vi "SCMP - Set Exp and Check FPS.vi"(6 "Andor":T1={"Handle"=0, "Pixel Encoding"="", "AOI Width"=0, "AOI Height"=0, "AOI Stride"=0, "Row Readout Time"=0.0, "Frame Readout Time"=0.0, "Interframe Time"=0.0, "Semaphore"=refnum, "SerialNumber"="", "Camera Model"="", "Controller ID"="", "Firmware Version"="", "Shutter"="Global", "BDiv"=1, "Time at Synch"=timestamp(3029526000.379448 s since 1904-01-01), "Idx"=0, "PreAmp"="", "Binning"=enum."1x1", "PixelReadoutRate"="", "Exposure (s)"=0.05, "Image Bytes"=0, "Image Pixels"=0, "SpuriousNoiseFilter"=FALSE, "Overlap"=FALSE, "CycleMode"=""} {"Exposure (s)" format="%^.3g"; "Time at Synch" format="%<%H:%M:%S>T"; "Interframe Time" format="%#_3g"; "Frame Readout Time" format="%_3g"; "Row Readout Time" format="%_3g"}, 7 "Set Exp or Check Fps (Set Exp)":enum16{"Set Exp", "Check FPS"}(ring), 8 "error in (no error)":errorcluster, 11 "Exposure [s]":dbl) -> (0 "error out":errorcluster, 3 "FPS":dbl=1.0)   [LabVIEW 2014]
doc: "Use this template to build a VI to use as a subVI."
uses:
  Camera/Andor Neo Info.ctl
  Controls/beaning.ctl
panel:
  out "FPS out":dbl=25.0 format="%.2f"
  out "Is Camera Exposure Acceptable":bool
  out "Maximum Exposure [ms]":dbl
  in  "FPS in":dbl=25.0 format="%0.2p"
  # "disabled"
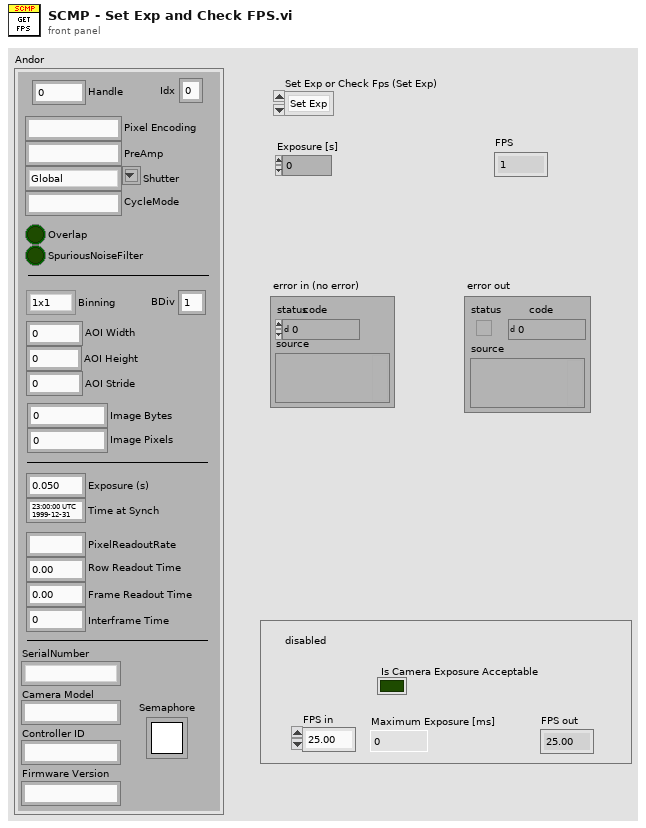
[diagram p1: front panel]
types:
  T1 = typedef "Andor Neo Info.ctl" = cluster{"Handle":i32, "Pixel Encoding":string, "AOI Width":i32, "AOI Height":i32, "AOI Stride":i32, "Row Readout Time":dbl, "Frame Readout Time":dbl, "Interframe Time":dbl, "Semaphore":T2, "SerialNumber":string, "Camera Model":string, "Controller ID":string, "Firmware Version":string, "Shutter":string, "BDiv":u8, "Time at Synch":timestamp, "Idx":i32, "PreAmp":string, "Binning":T3, "PixelReadoutRate":string, "Exposure (s)":dbl, "Image Bytes":i64, "Image Pixels":i64, "SpuriousNoiseFilter":bool, "Overlap":bool, "CycleMode":string}
  T2 = typedef "Semaphore RefNum" = refnum<k1>
  T3 = typedef "beaning.ctl" = enum16{"1x1", "2x2", "3x3", "4x4", "8x8"}
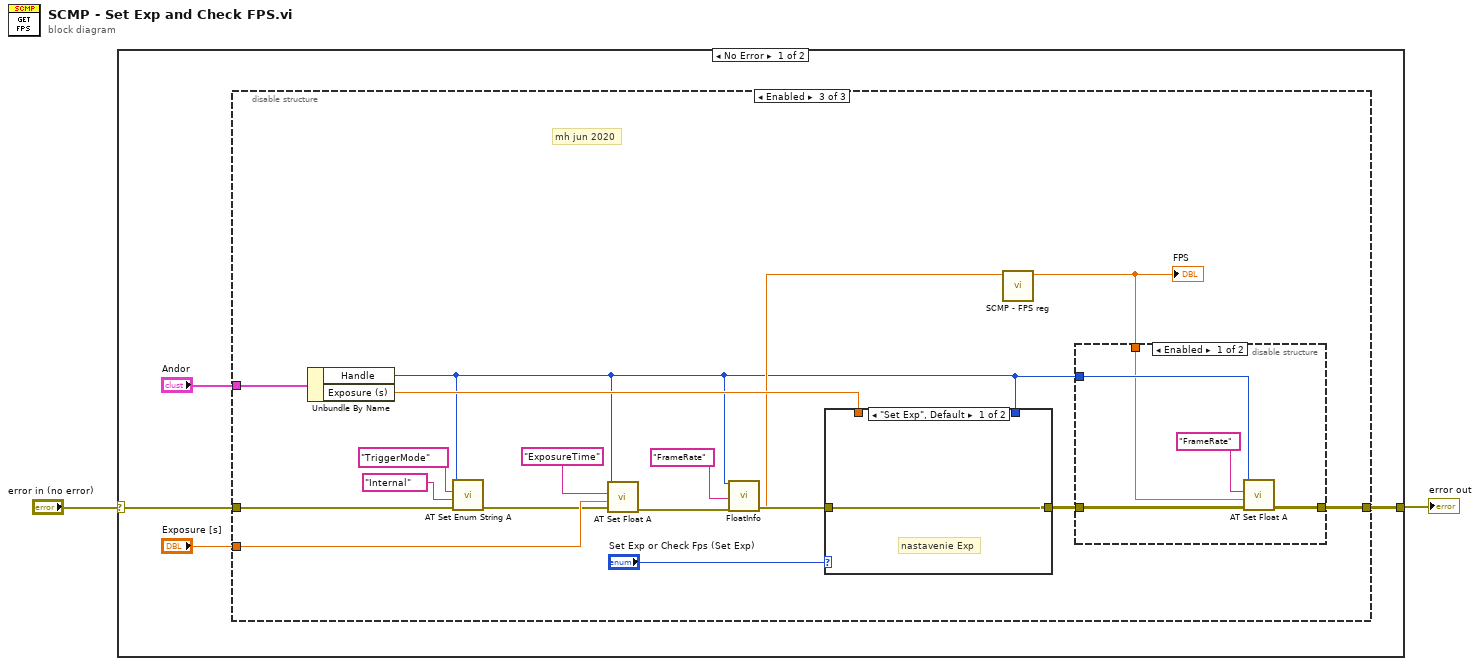
[diagram p0: block diagram]
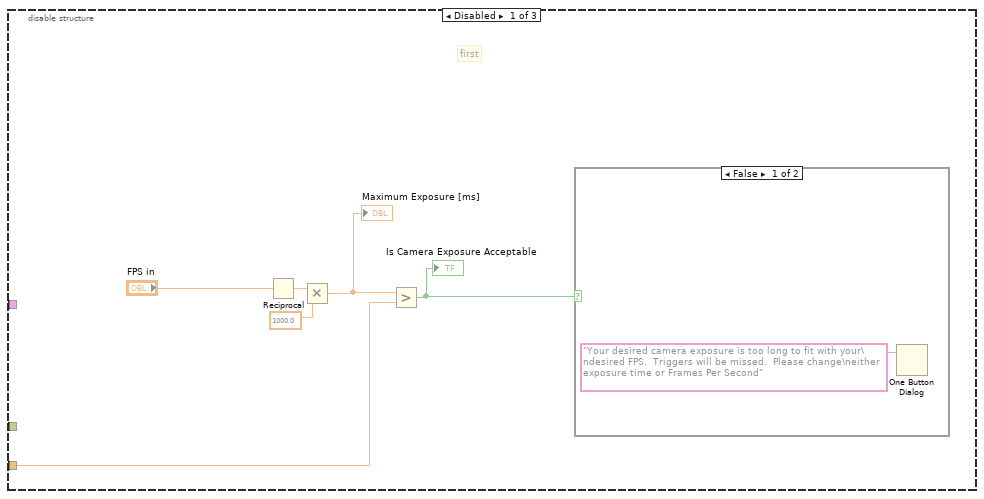
[diagram p2: hidden frame]
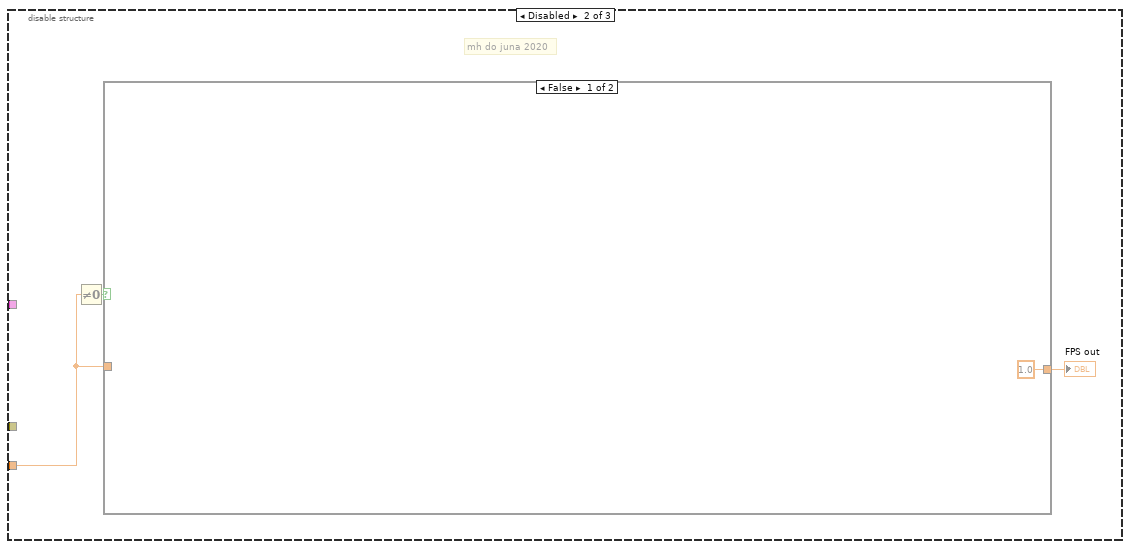
[diagram p4: hidden frame]
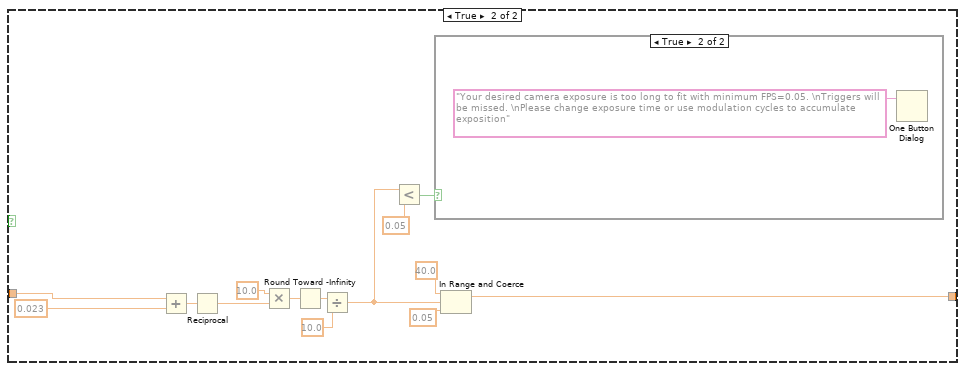
[diagram p5: hidden frame]
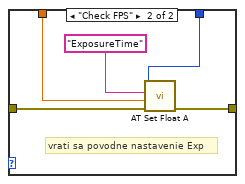
[diagram p8: hidden frame]
diagram:
  n1 = case shown="No Error" "error in (no error)" {
    selector: "error in (no error)" -> [w5 w62]
    tunnel: [w4 w62] -> w1
    frame No Error {
      n2 = disable-structure shown="Enabled" {
        disable-tunnel: "Exposure [s]" -> [w7 w15 w45]
        disable-tunnel: w5 -> [_ _ w36]
        disable-tunnel: [_ _ w41] -> w4
        disable-tunnel: "Andor" -> [_ _ w44]
        frame Disabled {
          # "first"
          n3 = Reciprocal(x="FPS in") -> (1/x=w11:dbl)
          n4 = Multiply(x=w11, y=1000.0) -> (x*y=w9:dbl)
          "Maximum Exposure [ms]" <- w9
          n5 = Greater?(x=w9, y=w7) -> (0:w8:bool)
          "Is Camera Exposure Acceptable" <- w8
          n6 = case shown="False" w8 {
            frame False {
              n7 = One Button Dialog(message="Your desired camera exposure is too long to fit with your\ndesired FPS.  Triggers will be missed.  Please change\neither exposure time or Frames Per Second") -> ()  [unwired: 1 in, 1 out]
            }
            frame True {
              # "Camera Exposure will fit between trigger pulses set by FPS"
            }
          }
        }
        frame Disabled {
          # "mh do juna 2020"
          n8 = Not Equal To 0?(x=w15) -> (x != 0?=w16:bool)
          n9 = case shown="False" w16 {
            tunnel: w15 -> [_ w31]
            tunnel: [1.0 ("upper limit") w18] -> w14
            frame False {
            }
            frame True {
              n10 = Add(x=w31, y=0.023) -> (x+y=w28:dbl)
              n11 = Reciprocal(x=w28) -> (1/x=w29:dbl)
              n12 = Multiply(x=10.0, y=w29) -> (x*y=w27:dbl)
              n13 = Round Toward -Infinity(1:w27) -> (0:w24:dbl)
              n14 = Divide(x=w24, y=10.0) -> (x/y=w19:dbl)
              n15 = Less?(x=w19, y=0.05) -> (x < y?=w20:bool)
              n16 = case shown="True" w20 {
                frame False {
                }
                frame True {
                  n17 = One Button Dialog(message="Your desired camera exposure is too long to fit with minimum FPS=0.05. \nTriggers will be missed. \nPlease change exposure time or use modulation cycles to accumulate exposition") -> ()  [unwired: 1 in, 1 out]
                }
              }
              n18 = In Range and Coerce(upper limit=40.0, x=w19, lower limit=0.05) -> (coerced(x)=w18:dbl)  [unwired: 1 out]
            }
          }
          "FPS out" <- w14
        }
        frame Enabled {
          # "mh jun 2020"
          n19 = Unbundle By Name(w44) -> ("Handle"=w34:i32, "Exposure (s)"=w43:dbl)
          n20 = call <userlib>:"AT Set Enum String A.vi"("error in (no error)"=w36, "String"="Internal" ("TriggerMode 2"), "Feature"="TriggerMode" ("Enum feature"), "Handle"=w34) -> ("error out"=w35:errorcluster)  [unwired: 6 in, 1 out]
          n21 = call <userlib>:"AT Set Float A.vi"("error in (no error)"=w35, "Value"=w45, "Feature"="ExposureTime", "Hndl"=w34) -> ("error out"=w48:errorcluster)  [unwired: 6 in, 1 out]
          n22 = call <userlib>:"FloatInfo.vi"("Handle"=w34, "Feature"="FrameRate", "error in (no error)"=w48) -> ("error out"=w46:errorcluster, "Max"=w39:dbl)  [unwired: 10 in, 5 out]
          n23 = case shown="\"Set Exp\", Default" "Set Exp or Check Fps (Set Exp)" {
            tunnel: w46 -> [w56 w61]
            tunnel: w43 -> [_ w59]
            tunnel: [w56 w58] -> w42
            tunnel: w34 -> [_ w57]
            frame "Set Exp", Default {
              # "nastavenie Exp"
            }
            frame "Check FPS" {
              # "vrati sa povodne nastavenie Exp"
              n24 = call <userlib>:"AT Set Float A.vi"("error in (no error)"=w61, "Value"=w59, "Feature"="ExposureTime", "Hndl"=w57) -> ("error out"=w58:errorcluster)  [unwired: 6 in, 1 out]
            }
          }
          n25 = call "SCMP - FPS reg.vi"("FPS in"=w39) -> ("FPS out"=w33:dbl)  [unwired: 10 in]
          "FPS" <- w33
          n26 = disable-structure shown="Enabled" {
            disable-tunnel: w42 -> [w54 w55]
            disable-tunnel: [w53 w55] -> w41
            disable-tunnel: w34 -> [w52 _]
            disable-tunnel: w33 -> [w50 _]
            frame Enabled {
              n27 = call <userlib>:"AT Set Float A.vi"("error in (no error)"=w54, "Value"=w50, "Feature"="FrameRate", "Hndl"=w52) -> ("error out"=w53:errorcluster)  [unwired: 6 in, 1 out]
            }
            frame Disabled {
            }
          }
        }
      }
    }
    frame Error {
    }
  }
  "error out" <- w1
